vi "building_timbre.vi"() -> ()   [LabVIEW 2022 SP3]
uses:
  <vilib>/express/express analysis/Spectral/Block/exnSpectralBlock spectral measurements RMS poly.vi
  <vilib>/express/express analysis/Spectral/Block/exnSpectralBlock spectral measurements RMS array WFM.vi
  <vilib>/express/express analysis/Spectral/Block/exnSpectralBlock spectral measurements RMS DDT.vi
  <vilib>/express/express analysis/Spectral/XNode/ExpressSpectralMeasurementsBlockNode.xnode
panel:
  in  "?":bool
  in  "?":bool
  in  "Audio File       Microphone":bool
  in  "Filter Type":string(combo)
  in  "Audio File":path
  in  "?":bool
  out "Input Signal":waveform(dbl)[](graph) caption="Data"
  out "Input Spectrum":cluster{"f0":dbl, "df":dbl, "magnitude":dbl[]}[](graph)
  in  "Duration of\nCollection (s)":dbl=1.0 caption="Duration (s)"
  out "Frequency of Note":dbl[](array[numeric]) format="%.2p"
  out "Note Detected":string
  in  "Run":bool
  in  "stop":bool
  in  "Array":T1(array[cluster])=[{"Freq"=214.28571428571428, "Amp"=8.22733603177593, "Wave Type"="Sine"}, {"Freq"=479.59183673469386, "Amp"=6.786888337237721, "Wave Type"="Sine"}, {"Freq"=704.0816326530612, "Amp"=7.041303382162077, "Wave Type"="Sine"}, {"Freq"=928.5714285714286, "Amp"=6.418172290569515, "Wave Type"="Sine"}, {"Freq"=61.224489795918366, "Amp"=0.19499801046990634, "Wave Type"="Sine"}] {"Amp" scale=0.0..10.0; "Freq" scale=0.0..1000.0}
  out "Generated Spectrum":dynamicdata(graph)
  out "Generated Signal":dynamicdata(graph) caption="Sine"
  # "Building Timbre"
  # "Input"
  # "Generated"
  # "Stop"
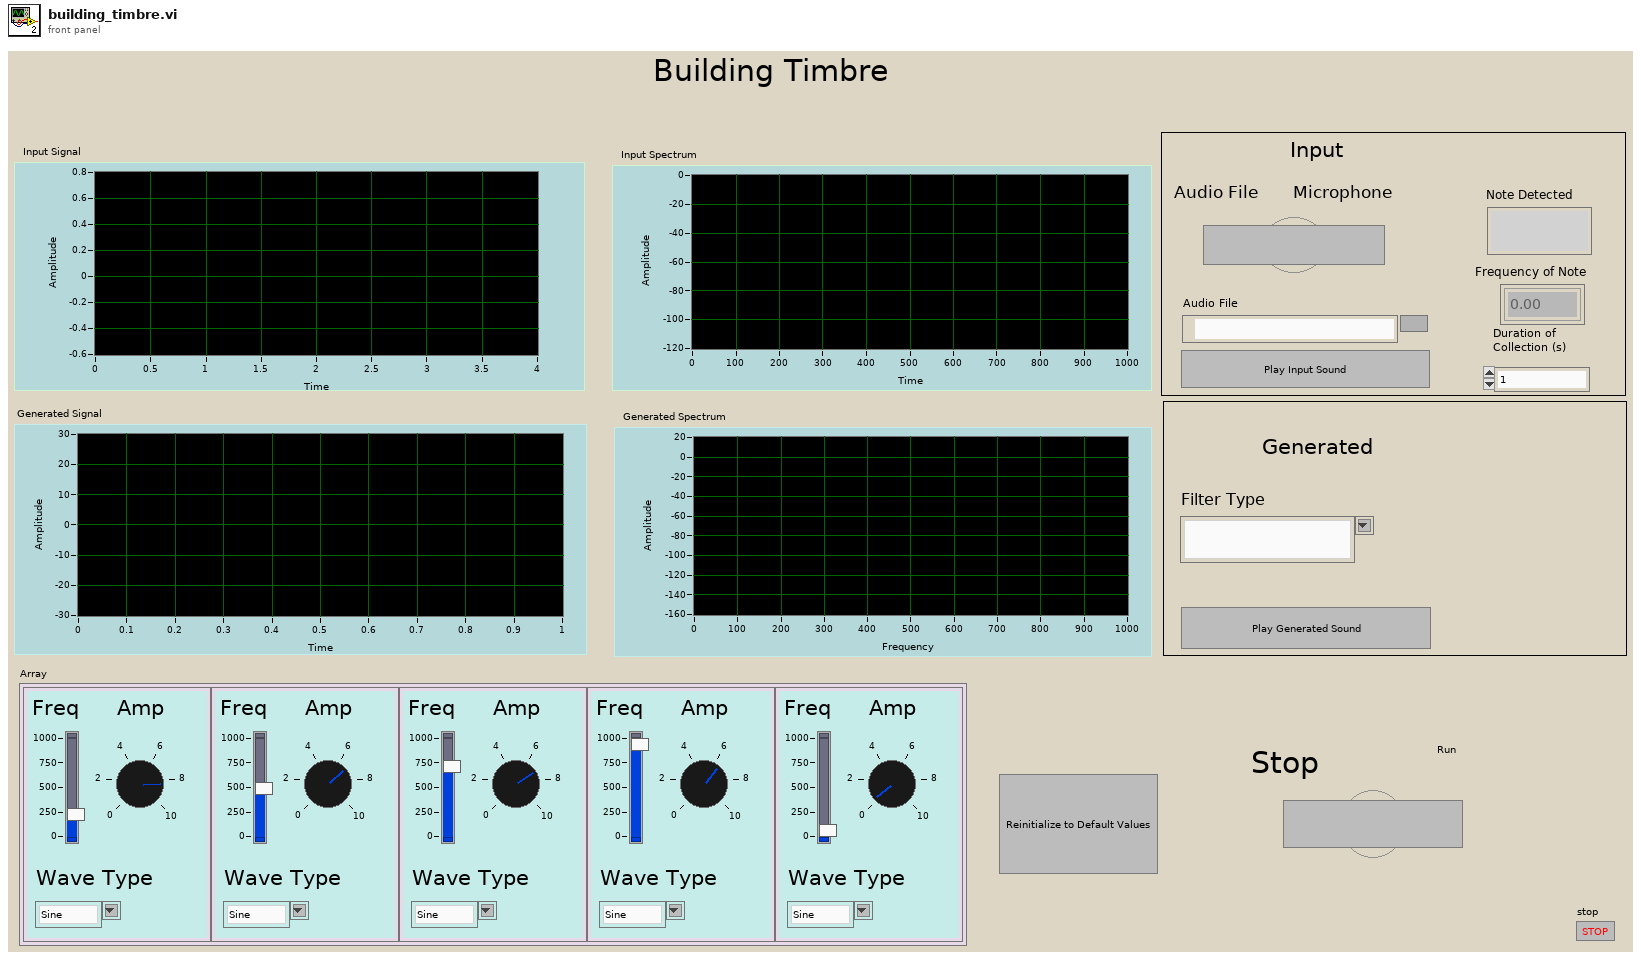
[diagram p1: front panel]
types:
  T1 = cluster{"Freq":dbl, "Amp":dbl, "Wave Type":string}[]
  T2 = cluster{"averaging mode":u16, "weighting mode":u16, "number of averages":u32}
  T3 = cluster{"dB On (F)":bool, "unwrap phase (F)":bool, "convert to degree (F)":bool}
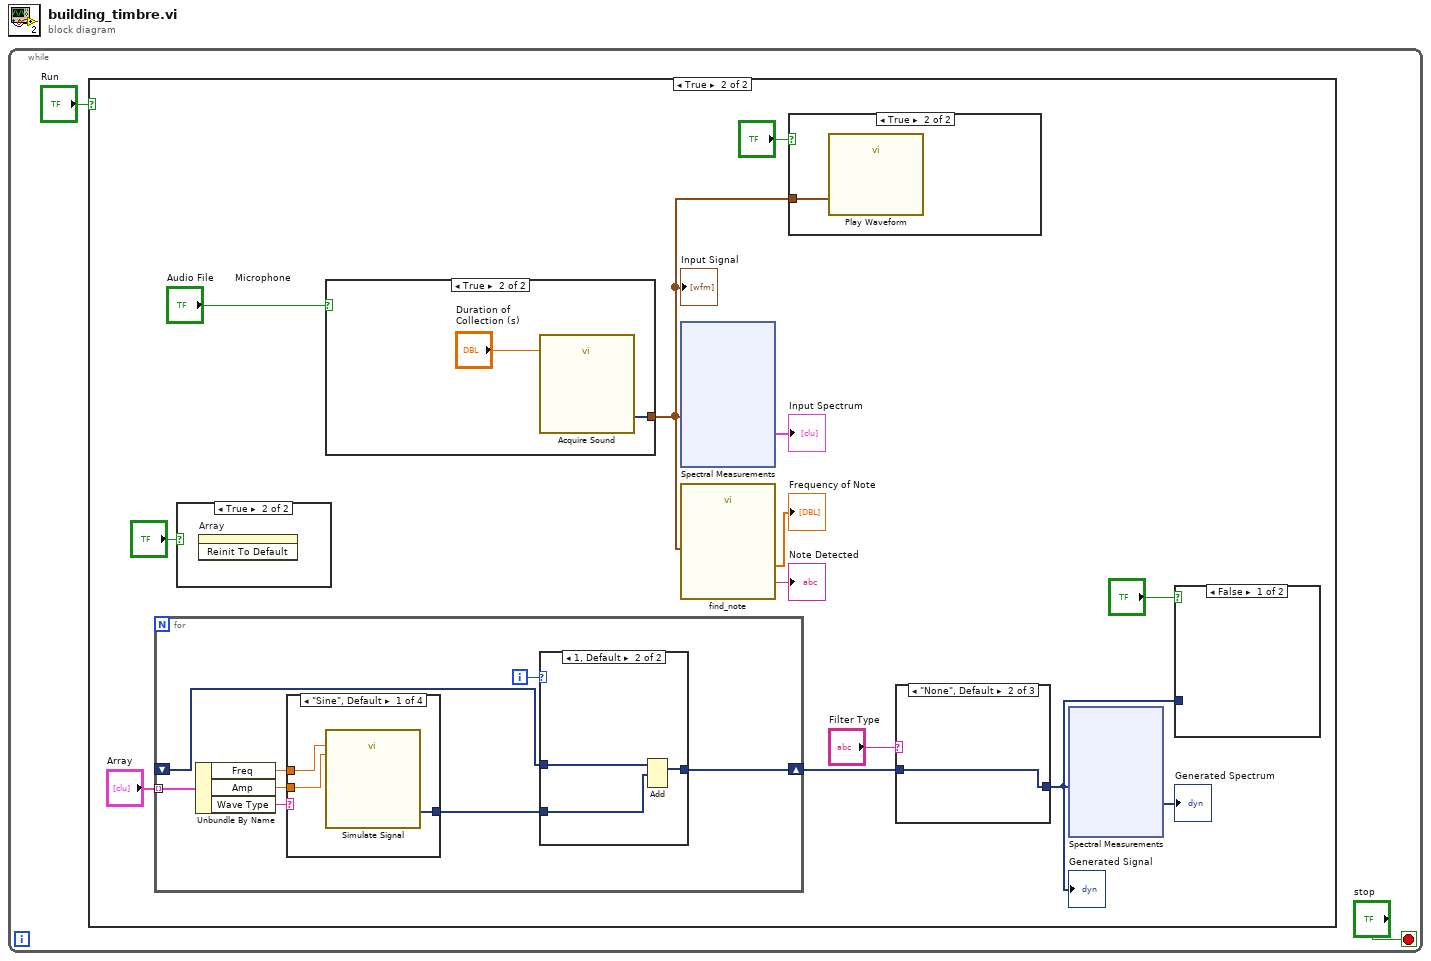
[diagram p0: block diagram]
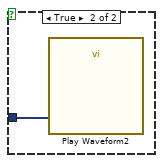
[diagram p4: hidden frame]
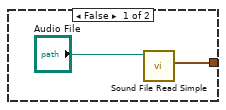
[diagram p5: hidden frame]
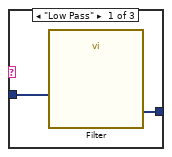
[diagram p6: hidden frame]
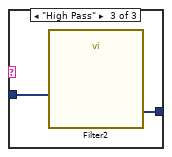
[diagram p7: hidden frame]
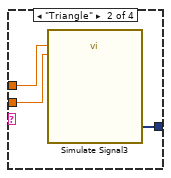
[diagram p9: hidden frame]
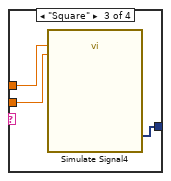
[diagram p10: hidden frame]
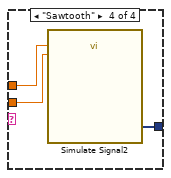
[diagram p11: hidden frame]
diagram:
  n1 = while {
    stop <- "stop" stop-if-true
    n2 = case shown="True" "Run" {
      frame False {
      }
      frame True {
        n3 = for {
          tunnel: "Array" -> [w30] mode=indexing
          shift-right: [w33] -> w7
          shift-left: _ -> [w32]
          i -> [w31]
          n4 = Unbundle By Name(w30) -> ("Freq"=w29:dbl, "Amp"=w28:dbl, "Wave Type"=w27:string)
          n5 = case shown="\"Sine\", Default" w27 {
            tunnel: [w35 w38 w41 w46] -> w34
            tunnel: w29 -> [w37 w39 w43 w45]
            tunnel: w28 -> [w36 w40 w42 w44]
            frame "Sine", Default {
              n6 = call "Simulate Signal"("Frequency"=w37, "Amplitude"=w36) -> ("Sine"=w35:dynamicdata)  [unwired: 12 in, 1 out]
            }
            frame "Triangle" {
              n7 = call "Simulate Signal3"("Frequency"=w39, "Amplitude"=w40) -> ("Triangle"=w38:dynamicdata)  [unwired: 12 in, 1 out]
            }
            frame "Square" {
              n8 = call "Simulate Signal4"("Frequency"=w43, "Amplitude"=w42) -> ("Square"=w41:dynamicdata)  [unwired: 12 in, 1 out]
            }
            frame "Sawtooth" {
              n9 = call "Simulate Signal2"("Frequency"=w45, "Amplitude"=w44) -> ("Sawtooth"=w46:dynamicdata)  [unwired: 12 in, 1 out]
            }
          }
          n10 = case shown="1, Default" w31 {
            tunnel: w34 -> [w47 w49]
            tunnel: [w47 w48] -> w33
            tunnel: w32 -> [_ w50]
            frame 0 {
            }
            frame 1, Default {
              n11 = Add(1:w49, 2:w50) -> (0:w48:dynamicdata)  [unwired: 1 in, 1 out]
            }
          }
        }
        n12 = case shown="True" "?" {
          frame False {
          }
          frame True {
            n13 = invoke on="Array" class="Arr (strict)" method="Reinit To Default"() -> ()  [unwired: 3 in, 3 out]
          }
        }
        n14 = case shown="True" "Audio File       Microphone" {
          tunnel: [w17 w19] -> w8
          frame False {
            n15 = call <vilib>:"Sound File Read Simple.vi"("path"="Audio File") -> ("data"=w17:waveform(dbl)[])  [unwired: 7 in, 3 out]
          }
          frame True {
            n16 = call "Acquire Sound"("Duration (s)"="Duration of\nCollection (s)") -> ("Data"=w19:dynamicdata)  [unwired: 17 in, 1 out]
          }
        }
        "Input Signal" <- w8
        n17 = xnode "Spectral Measurements"("Signals"=w8) -> ("FFT - (RMS)"=→"Input Spectrum":cluster{"f0":dbl, "df":dbl, "magnitude":dbl[]}[])  [unwired: 1 in, 2 out]
        n18 = call "find_note.vi"("Data"=w8) -> ("Note"=→"Note Detected":string, "Frequency"=→"Frequency of Note":dbl[])  [unwired: 9 in]
        n19 = case shown="True" "?" {
          tunnel: w8 -> [_ w26]
          frame False {
          }
          frame True {
            n20 = call "Play Waveform"("Data"=w26) -> ()  [unwired: 18 in, 1 out]
          }
        }
        n21 = case shown="\"None\", Default" "Filter Type" {
          tunnel: w7 -> [w22 w23 w25]
          tunnel: [w21 w23 w24] -> w5
          frame "Low Pass" {
            n22 = call "Filter"("Signal"=w22) -> ("Filtered Signal"=w21:dynamicdata)  [unwired: 9 in, 1 out]
          }
          frame "None", Default {
          }
          frame "High Pass" {
            n23 = call "Filter2"("Signal"=w25) -> ("Filtered Signal"=w24:dynamicdata)  [unwired: 9 in, 1 out]
          }
        }
        "Generated Signal" <- w5
        n24 = xnode "Spectral Measurements"("Signals"=w5) -> ("FFT - (RMS)"=→"Generated Spectrum":dynamicdata)  [unwired: 1 in, 2 out]
        n25 = case shown="False" "?" {
          tunnel: w5 -> [_ w16]
          frame False {
          }
          frame True {
            n26 = call "Play Waveform2"("Data"=w16) -> ()  [unwired: 18 in, 1 out]
          }
        }
      }
    }
  }
